vi "Wrap Actor.vi"() -> ()   [LabVIEW 2020, in "Wrapped Actor.lvlib"]
uses:
  Wrapped Actor.lvlib
  Data Message/Data Message.lvclass
  Data Message/Data Message.lvclass/Data Message.ctl
  93fa84f4-be94-473d-99fc-dbd7b0327947.vi
  Data Message/Read Value.vi
  <vilib>/Comparison/Equal/Equal Functor/Equal Functor.lvclass
  Wrapper/Wrapper.lvclass
panel:
  in  "stop":bool
  out "Waveform Chart":dbl[][](graph)
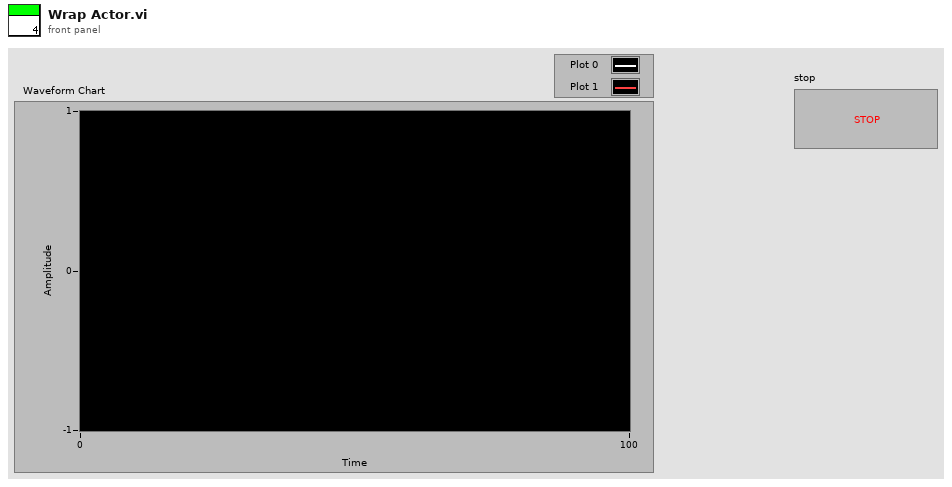
[diagram p1: front panel]
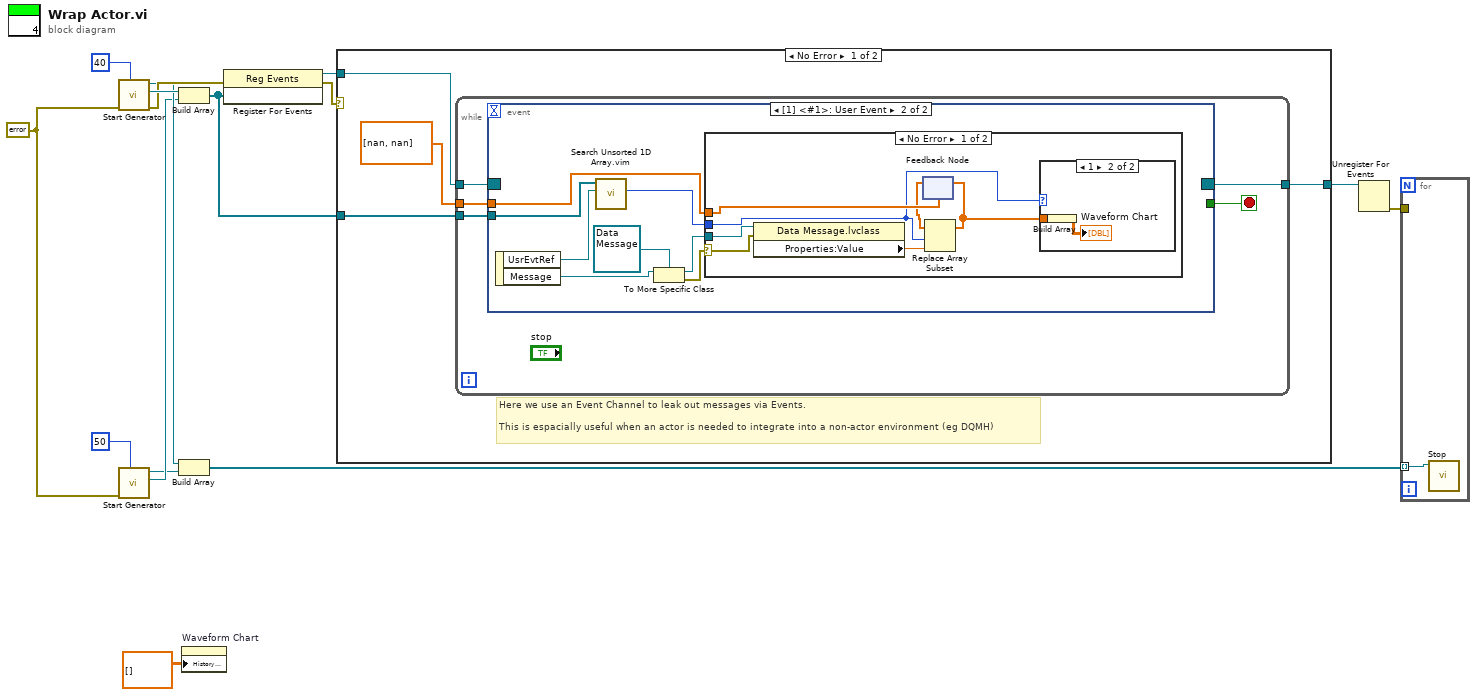
[diagram p0: block diagram]
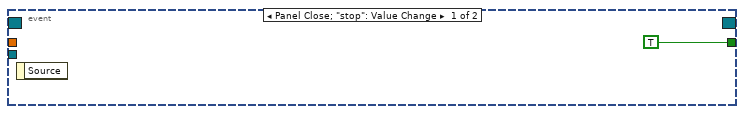
[diagram p2: hidden frame]
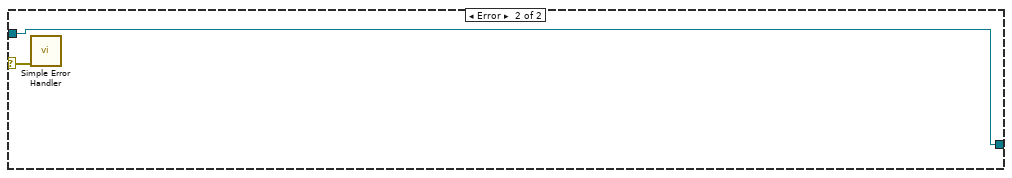
[diagram p5: hidden frame]
diagram:
  w9 = errorcluster {"status"=FALSE, "code"=0, "source"=""} ("error in (no error)")
  n1 = call "Start Generator.vi"("Timeout ms"=40, "error in (no error)"=w9) -> ("error out"=w12:errorcluster, "New Message Event"=w13:refnum<user-event>, "Wrapper out"=w10:refnum<class "Wrapper.lvclass">)  [unwired: 7 in]
  n2 = call "Start Generator.vi"("Timeout ms"=50, "error in (no error)"=w9) -> ("New Message Event"=w8:refnum<user-event>, "Wrapper out"=w6:refnum<class "Wrapper.lvclass">)  [unwired: 7 in, 1 out]
  n3 = Build Array(w13, w8) -> (w7:refnum<user-event>[])
  n4 = Build Array(w10, w6) -> (w5:refnum<class "Wrapper.lvclass">[])
  n5 = property on="Waveform Chart" class="WFChart (strict)"("History Data"=dbl[][] []) -> ()  [unwired: 2 in, 2 out]
  n6 = register-events(error in=w12, w7) -> (reference out=w15:refnum<event-registration>, error out=w14:errorcluster)  [unwired: 1 in]
  n7 = case shown="No Error" w14 {
    selector: w14 -> [_ w44]
    tunnel: w15 -> [w19 w43]
    tunnel: [w18 w43] -> w11
    tunnel: w7 -> [w17 _]
    frame No Error {
      # "Here we use an Event Channel to leak out messages via Events.\n\nThis is espacially useful when an actor is needed to integrate into a non-actor environment (eg DQMH)"
      n8 = while {
        tunnel: w19 -> [w24]
        tunnel: [w22] -> w18
        tunnel: w17 -> [w21]
        tunnel: dbl[] [nan, nan] ("Properties:Value") -> [w20]
        stop <- w23 stop-if-true
        n9 = event shown="[1] <#1>: User Event" {
          selector: w24 -> [_ _]
          dyn-events: [_ _] -> w22
          timeout: _ -> [_ _]
          tunnel: [TRUE _] -> w23
          tunnel: w21 -> [_ w29]
          tunnel: w20 -> [_ w27]
          event Panel Close; "stop": Value Change {
            n10 = event-data() -> ()  [unwired: 1 in, 1 out]
          }
          event User Event {
            n11 = event-data() -> ("UsrEvtRef"=w28:refnum<user-event>, "Message"=w33:refnum<class "Message.lvclass">)  [unwired: 1 in]
            n12 = call "Search Unsorted 1D Array.vim"("element"=w28, "unsorted 1D array"=w29) -> ("index of element"=w26:i32)  [unwired: 9 in]
            n13 = To More Specific Class(target class=refnum<class "Data Message.lvclass"> refnum ("Wrapped Actor.lvlib:Data Message.lvclass"), reference=w33) -> (specific class reference=w30:refnum<class "Data Message.lvclass">, error out=w31:errorcluster)  [unwired: 1 in]
            n14 = case shown="No Error" w31 {
              selector: w31 -> [w40 _]
              tunnel: w30 -> [w39 _]
              tunnel: w27 -> [w37 _]
              tunnel: w26 -> [w35 _]
              frame No Error {
                n15 = property class="Data Message.lvclass"(reference=w39, error in=w40) -> ("Properties:Value"=w38:dbl)  [unwired: 2 out]
                n16 = feedback #1(w37) -> (w36:dbl[])
                n17 = Replace Array Subset(array=w36, new element=w38, index=w35) -> (w34:dbl[])
                n18 = feedback-in #1(w34) -> ()
                n19 = case shown="1" w35 {
                  tunnel: w34 -> [_ w42]
                  frame 0, Default {
                  }
                  frame 1 {
                    n20 = Build Array(w42) -> (→"Waveform Chart":dbl[][])
                  }
                }
              }
              frame Error {
              }
            }
          }
        }
      }
    }
    frame Error {
      n21 = call <vilib>:"Simple Error Handler.vi"("error in (no error)"=w44) -> ()  [unwired: 4 in, 5 out]
    }
  }
  n22 = Unregister For Events(event registration refnum=w11) -> (error out=w4:errorcluster)  [unwired: 1 in]
  n23 = for {
    tunnel: w5 -> [w45] mode=indexing
    tunnel: w4 -> [_]
    n24 = call "Stop.vi"("Wrapper in"=w45) -> ()  [unwired: 9 in, 2 out]
  }
